vi "String to I32.vi"(8 "error in":errorcluster, 11 "Integer String":string) -> (0 "error out":errorcluster, 3 "I32":i32)   [LabVIEW 2024, in "Electronic Datasheet.lvlib"]
doc: "Converts the string representation of a number in a specified base to an equivalent 32-bit signed integer."
uses:
  Core/Electronic Datasheet.lvlib
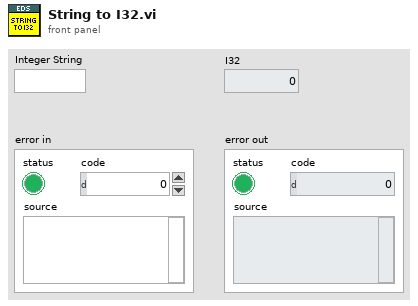
[diagram p1: front panel]
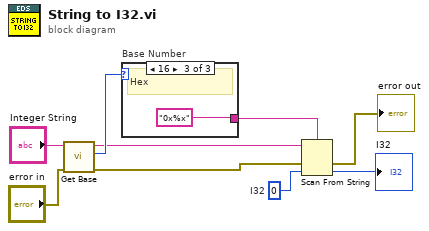
[diagram p0: block diagram]
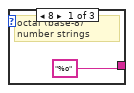
[diagram p2: hidden frame]
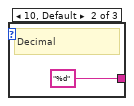
[diagram p3: hidden frame]
diagram:
  w7 = 0  # I32
  n1 = call "Get Base.vi"("error in"="error in", "Default Value"="Integer String") -> ("error out"=w1:errorcluster, "Number Base"=w8:u8, "Default Value (dup)"=w5:string)  [unwired: 7 in]
  n2 = case "Base Number" shown="16" w8 {
    tunnel: ["%o" ("format string") "%d" ("format string") "0x%x" ("format string")] -> w6
    frame 8 {
      # "octal (base-8) number strings"
    }
    frame 10, Default {
      # "Decimal"
    }
    frame 16 {
      # "Hex"
    }
  }
  n3 = Scan From String(format string=w6, input string=w5, error in=w1, default 1=w7) -> (error out=→"error out":errorcluster, output 1=→"I32":i32)  [unwired: 1 in, 2 out]
